vi "HandleClapper.vi"(7 "InitState":T1=enum."Out", 8 "error in (no error)":errorcluster, 10 "ClapperOut":bool, 11 "ClapperIn":bool) -> (0 "error out":errorcluster, 3 "State":T1=enum."Middle")   [LabVIEW 2015]
doc: "Switches the clapper state. if ClapperIn is true, it shifts the state one inward (in -> in, middle -> in, out -> middle). If ClapperOut is true, shifts the state one outward (in -> middle, middle -> out, out -> out)."
uses:
  DoubleSolenoidAction.ctl
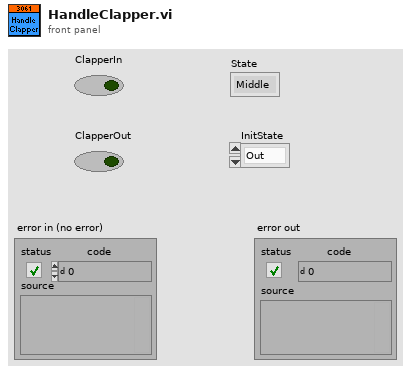
[diagram p1: front panel]
types:
  T1 = typedef "DoubleSolenoidAction.ctl" = enum16{"Init", "Middle", "In", "Out"}
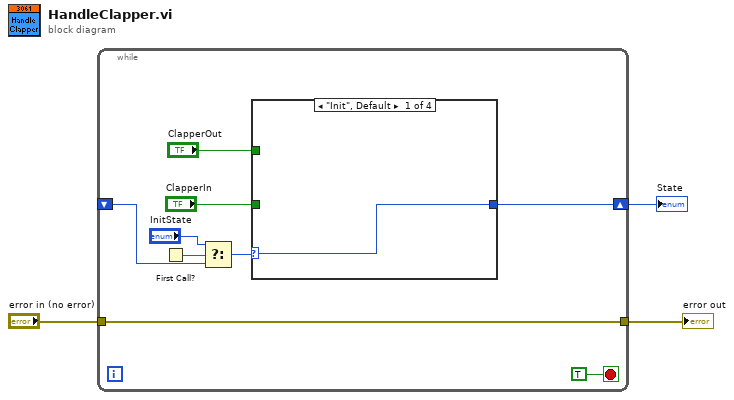
[diagram p0: block diagram]
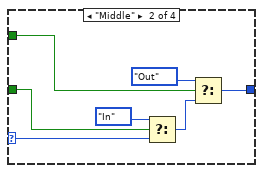
[diagram p2: hidden frame]
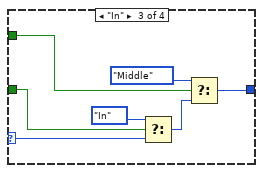
[diagram p3: hidden frame]
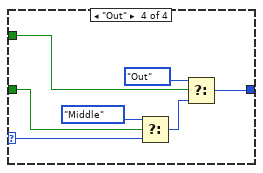
[diagram p4: hidden frame]
diagram:
  n1 = while {
    shift-right: [w12] -> w3
    shift-left: _ -> [w5]
    tunnel: "error in (no error)" -> [w9]
    tunnel: [w9] -> w1
    stop <- TRUE stop-if-true
    n2 = First Call?() -> (First Call?: T/F=w6:bool)
    n3 = Select(t="InitState", s=w6, f=w5) -> (s? t:f=w4:T1)
    n4 = case shown="\"Init\", Default" w4 {
      selector: w4 -> [w13 w20 w23 w31]
      tunnel: [w13 w17 w24 w30] -> w12
      tunnel: "ClapperOut" -> [_ w14 w21 w29]
      tunnel: "ClapperIn" -> [_ w15 w22 w28]
      frame "Init", Default {
      }
      frame "Middle" {
        n5 = Select(t=DoubleSolenoidAction."In", s=w15, f=w20) -> (s? t:f=w18:T1)
        n6 = Select(t=DoubleSolenoidAction."Out", s=w14, f=w18) -> (s? t:f=w17:T1)
      }
      frame "In" {
        n7 = Select(t=DoubleSolenoidAction."In", s=w22, f=w23) -> (s? t:f=w26:T1)
        n8 = Select(t=DoubleSolenoidAction."Middle", s=w21, f=w26) -> (s? t:f=w24:T1)
      }
      frame "Out" {
        n9 = Select(t=DoubleSolenoidAction."Middle", s=w28, f=w31) -> (s? t:f=w33:T1)
        n10 = Select(t=DoubleSolenoidAction."Out", s=w29, f=w33) -> (s? t:f=w30:T1)
      }
    }
  }
  "State" <- w3
  "error out" <- w1
